vi "ParseColor.vi"(3 "HTML in":string) -> (1 "Color":u32(colorbox))   [LabVIEW 2015]
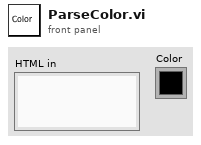
[diagram p1: front panel]
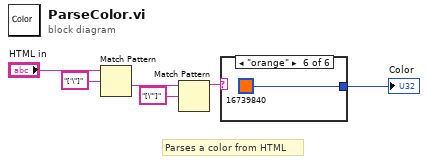
[diagram p0: block diagram]
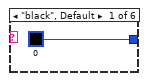
[diagram p2: hidden frame]
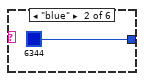
[diagram p3: hidden frame]
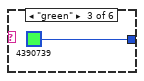
[diagram p4: hidden frame]
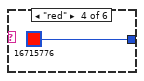
[diagram p5: hidden frame]
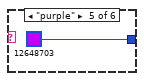
[diagram p6: hidden frame]
diagram:
  # "Parses a color from HTML"
  n1 = Match Pattern(string="HTML in", regular expression="['\"]" ("search string/char (-)")) -> (after substring=w4:string)  [unwired: 1 in, 3 out]
  n2 = Match Pattern(string=w4, regular expression="[\"']" ("search string/char (-)")) -> (before substring=w2:string)  [unwired: 1 in, 3 out]
  n3 = case shown="\"orange\"" w2 {
    tunnel: [u32 0 ("Color") u32 6344 ("Color") u32 4390739 ("Color") u32 16715776 ("Color") u32 12648703 ("Color") u32 16739840 ("Color")] -> w6
    frame "black", Default {
    }
    frame "blue" {
    }
    frame "green" {
    }
    frame "red" {
    }
    frame "purple" {
    }
    frame "orange" {
    }
  }
  "Color" <- w6
